vi "读D协议转字符.vi"(10 "读取D个数":i32=1 min=0 max=10, 11 "读取D地址":i32) -> (2 "读取的字节数":i32, 3 "连接的字符串":string)   [LabVIEW 2018]
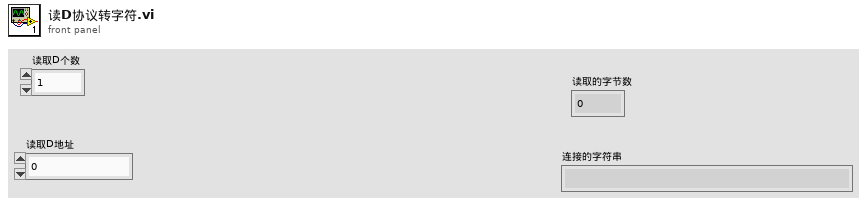
[diagram p1: front panel]
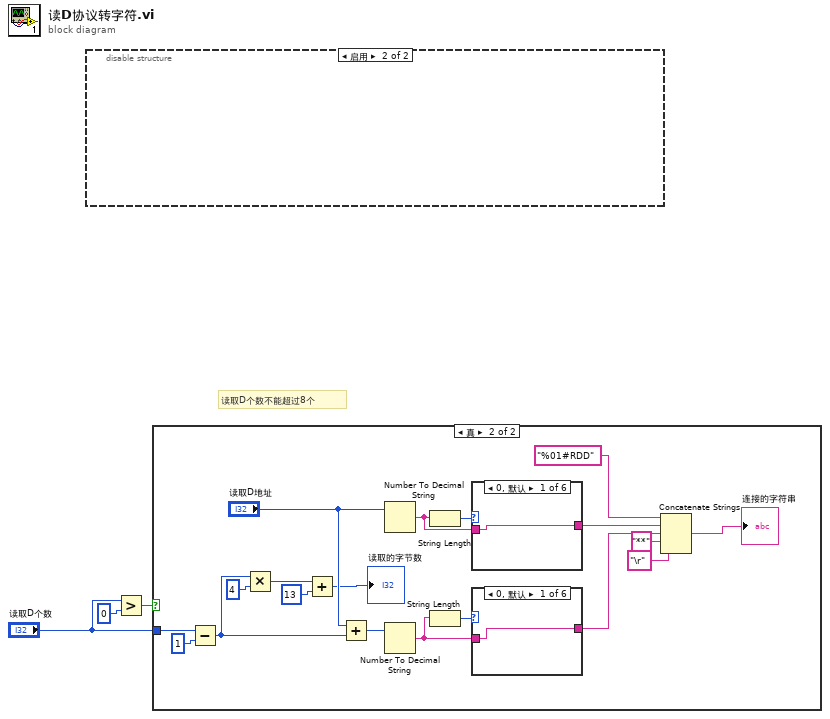
[diagram p0: block diagram]
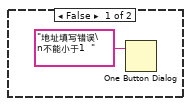
[diagram p2: hidden frame]
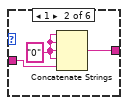
[diagram p3: hidden frame]
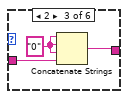
[diagram p4: hidden frame]
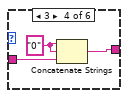
[diagram p5: hidden frame]
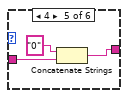
[diagram p6: hidden frame]
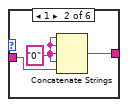
[diagram p8: hidden frame]
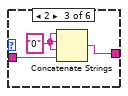
[diagram p9: hidden frame]
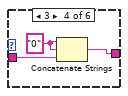
[diagram p10: hidden frame]
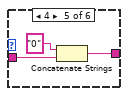
[diagram p11: hidden frame]
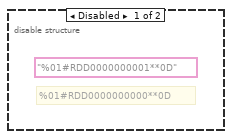
[diagram p13: hidden frame]
diagram:
  # "读取D个数不能超过8个"
  n1 = disable-structure shown="启用" {
    frame Disabled {
      (unwired) "%01#RDD0000000001**0D" ("字符串")
      # "%01#RDD0000000000**0D"
    }
    frame Enabled {
    }
  }
  n2 = Greater?(x="读取D个数", y=0) -> (0:w2:bool)
  n3 = case shown="真" w2 {
    tunnel: "读取D个数" -> [_ w8]
    frame False {
      n4 = One Button Dialog(message="地址填写错误\n不能小于1  " ("消息")) -> ()  [unwired: 1 in, 1 out]
    }
    frame True {
      n5 = Subtract(x=w8, y=1) -> (x-y=w7:i32)
      n6 = Multiply(x=w7, y=4) -> (x*y=w15:i32)
      n7 = Add(x=w15, y=13) -> (x+y=→"读取的字节数":i32)
      n8 = Add(x="读取D地址", y=w7) -> (x+y=w18:i32)
      n9 = Number To Decimal String(number="读取D地址") -> (decimal integer string=w14:string)  [unwired: 1 in]
      n10 = Number To Decimal String(number=w18) -> (decimal integer string=w20:string)  [unwired: 1 in]
      n11 = String Length(string=w14) -> (length=w13:i32)
      n12 = String Length(string=w20) -> (length=w19:i32)
      n13 = case shown="0, 默认" w13 {
        tunnel: w14 -> [w38 w41 w44 w47 w50 w51]
        tunnel: [w38 w39 w42 w45 w48 w51] -> w22
        frame 0, Default {
        }
        frame 1 {
          w40 = "0" ("字符串")
          n14 = Concatenate Strings(w40, w40, w40, w40, w41) -> (w39:string)
        }
        frame 2 {
          w43 = "0" ("字符串")
          n15 = Concatenate Strings(w43, w43, w43, w44) -> (w42:string)
        }
        frame 3 {
          w46 = "0" ("字符串")
          n16 = Concatenate Strings(w46, w46, w47) -> (w45:string)
        }
        frame 4 {
          n17 = Concatenate Strings("0" ("字符串"), w50) -> (w48:string)
        }
        frame 5 {
        }
      }
      n18 = case shown="0, 默认" w19 {
        tunnel: w20 -> [w24 w27 w30 w33 w36 w37]
        tunnel: [w24 w25 w28 w31 w34 w37] -> w23
        frame 0, Default {
        }
        frame 1 {
          w26 = "0" ("字符串")
          n19 = Concatenate Strings(w26, w26, w26, w26, w27) -> (w25:string)
        }
        frame 2 {
          w29 = "0" ("字符串")
          n20 = Concatenate Strings(w29, w29, w29, w30) -> (w28:string)
        }
        frame 3 {
          w32 = "0" ("字符串")
          n21 = Concatenate Strings(w32, w32, w33) -> (w31:string)
        }
        frame 4 {
          n22 = Concatenate Strings("0" ("字符串"), w36) -> (w34:string)
        }
        frame 5 {
        }
      }
      n23 = Concatenate Strings("%01#RDD" ("字符串"), w22, w23, "**" ("字符串"), "\r" ("字符串")) -> (→"连接的字符串":string)
    }
  }
